vi "removezeroes.vi"(8 "index":dbl[](array[numeric]), 11 "B":dbl[](array[numeric])) -> (0 "index out":dbl[](array[numeric]), 3 "B out":dbl[](array[numeric]))   [LabVIEW 2015]
panel:
  in  "doof":dbl[](array[numeric])
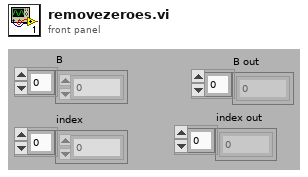
[diagram p1: front panel]
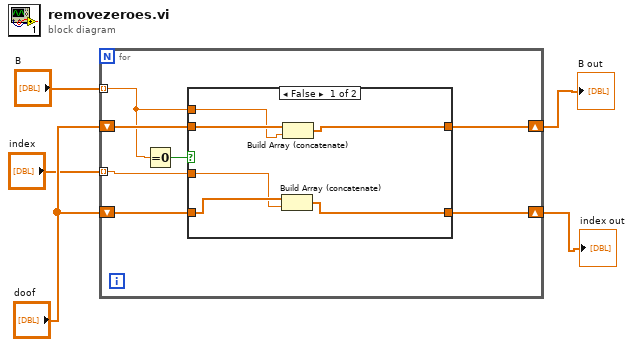
[diagram p0: block diagram]
diagram:
  n1 = for {
    shift-right: [w9] -> w1
    shift-left: "doof" -> [w8]
    shift-right: [w11] -> w2
    shift-left: "doof" -> [w10]
    tunnel: "B" -> [w7] mode=indexing
    tunnel: "index" -> [w6] mode=indexing
    n2 = Equal To 0?(x=w7) -> (x = 0?=w12:bool)
    n3 = case shown="False" w12 {
      tunnel: [w14 w20] -> w11
      tunnel: w10 -> [w18 w20]
      tunnel: [w13 w19] -> w9
      tunnel: w8 -> [w17 w19]
      tunnel: w7 -> [w16 _]
      tunnel: w6 -> [w15 _]
      frame False {
        n4 = Build Array (concatenate)(w17, w15) -> (w13:dbl[])
        n5 = Build Array (concatenate)(w18, w16) -> (w14:dbl[])
      }
      frame True {
      }
    }
  }
  "B out" <- w2
  "index out" <- w1
